vi "SaveProject.vi"(8 "error in (no error)":errorcluster, 9 "XML File Path":path, 10 "BrowerComponent":refnum<class "BrowerComponent.lvclass">, 11 "XML Project":refnum<class "XML Project.lvclass">) -> (0 "error out":errorcluster, 3 "ProjectManager out":refnum<class "XML Project.lvclass">)   [LabVIEW 2015, in "XML Project.lvclass"]
uses:
  XML Project.lvclass
  Brower Console/Models/BrowerComponent/BrowerComponent/BrowerComponent.lvclass
  <vilib>/NI/AQ Character Lineator/JSON Serializer/JSON Serializer.lvclass
  <vilib>/Utility/xml.llb/Write to XML File(string).vi
  <vilib>/NI/AQ Character Lineator/Serializer/Serializer.lvclass
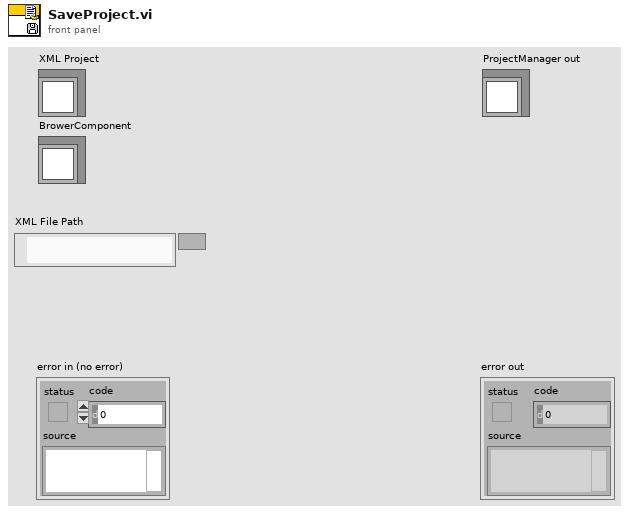
[diagram p1: front panel]
types:
  T1 = enum16{"open", "replace", "create", "open or create", "replace or create", "replace or create with confirmation"}
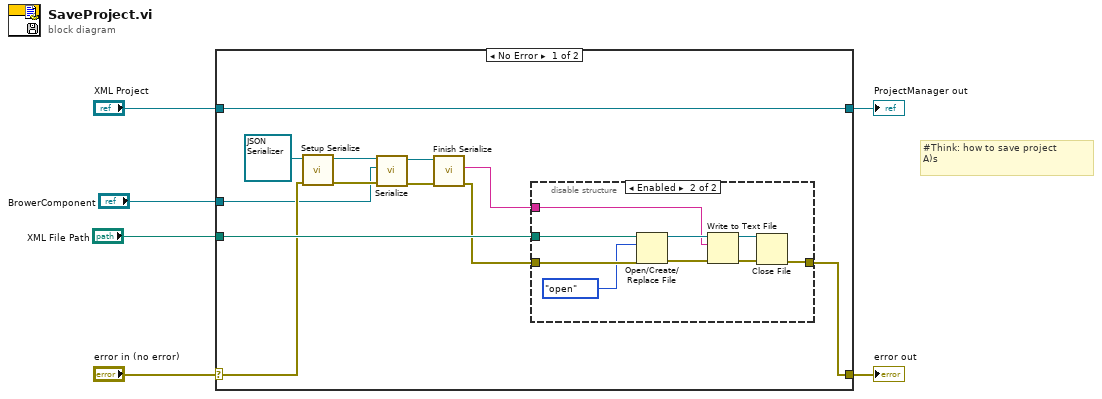
[diagram p0: block diagram]
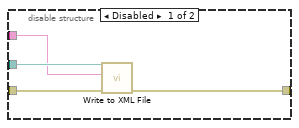
[diagram p2: hidden frame]
diagram:
  # "#Think: how to save project \nA)s"
  n1 = case shown="No Error" "error in (no error)" {
    selector: "error in (no error)" -> [w15 w33]
    tunnel: [w8 w33] -> w5
    tunnel: [w18 w32] -> w3
    tunnel: "XML Project" -> [w18 w32]
    tunnel: "BrowerComponent" -> [w12 _]
    tunnel: "XML File Path" -> [w17 _]
    frame No Error {
      n2 = call <vilib>:"Setup Serialize.vi"("error in (no error)"=w15, "Serializer in"=refnum<class "JSON Serializer.lvclass"> refnum ("JSON Serializer.lvclass")) -> ("error out"=w13:errorcluster, "Serializer out"=w14:refnum<class "JSON Serializer.lvclass">)  [unwired: 8 in]
      n3 = call-dynamic "Serialize.vi"("error in (no error)"=w13, "Serializable"=w12, "JSON Serializer in"=w14) -> ("error out"=w10:errorcluster, "JSON Serializer out"=w11:refnum<class "JSON Serializer.lvclass">)  [unwired: 7 in]
      n4 = call <vilib>:"Finish Serialize.vi"("error in (no error)"=w10, "Serializer in"=w11) -> ("error out"=w9:errorcluster, "String"=w7:string)  [unwired: 6 in, 2 out]
      n5 = disable-structure shown="Enabled" {
        disable-tunnel: w17 -> [w22 w31]
        disable-tunnel: w7 -> [w21 w24]
        disable-tunnel: w9 -> [w20 w30]
        disable-tunnel: [w19 w25] -> w8
        frame Disabled {
          n6 = call-poly <vilib>:"Write to XML File.vi"("error in (no error)"=w20, "XML Input"=w21, "XML File Path"=w22) -> ("error out"=w19:errorcluster)  [unwired: 6 in, 2 out]
        }
        frame Enabled {
          n7 = Open/Create/Replace File(file path (use dialog)=w31, error in=w30, operation (0:open)=T1."open") -> (refnum out=w29:refnum<file>, error out=w28:errorcluster)  [unwired: 3 in, 1 out]
          n8 = Write to Text File(file (use dialog)=w29, text=w24, error in=w28) -> (refnum out=w26:refnum<file>, error out=w27:errorcluster)  [unwired: 1 in, 1 out]
          n9 = Close File(refnum=w26, error in=w27) -> (error out=w25:errorcluster)  [unwired: 1 out]
        }
      }
    }
    frame Error {
    }
  }
  "error out" <- w5
  "ProjectManager out" <- w3
